vi "set_config_cluster.vi"(8 "error in (no error)":errorcluster, 10 "config cluster variant":variant, 11 "ClockDL090202FPGA in":refnum<class "ClockDL090202FPGA.lvclass">) -> (0 "error out":errorcluster, 3 "ClockDL090202FPGA out":refnum<class "ClockDL090202FPGA.lvclass">)   [LabVIEW 2010, in "ClockDL090202FPGA.lvclass"]
uses:
  ClockDL090202FPGA.lvclass
  ClockDL090202FPGA.lvclass/ClockDL090202FPGA.ctl
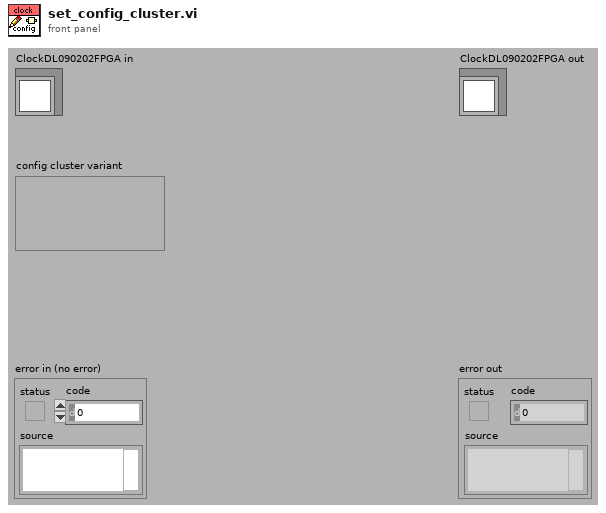
[diagram p1: front panel]
types:
  T1 = typedef "ClockDL090202FPGA.lvclass/config_data_cluster.ctl" = cluster{"FPGAWrapper":T2, "type":T3}
  T2 = typedef "plugin_specification.ctl" = cluster{"class path":string, "configuration":string, "label":string, "settings name":string}
  T3 = typedef "ClockDL090202FPGA.lvclass/type_enum.ctl" = enum16{"pixel clock", "gate 1", "gate 2", "gate 3"}
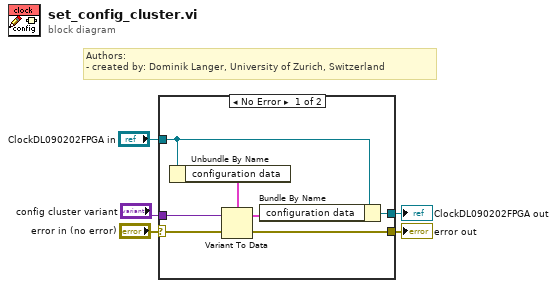
[diagram p0: block diagram]
diagram:
  # "Authors: \n- created by: Dominik Langer, University of Zurich, Switzerland"
  n1 = case shown="No Error" "error in (no error)" {
    selector: "error in (no error)" -> [w6 w14]
    tunnel: "config cluster variant" -> [w11 _]
    tunnel: "ClockDL090202FPGA in" -> [w10 w13]
    tunnel: [w8 w14] -> w3
    tunnel: [w7 w13] -> w2
    frame No Error {
      n2 = Unbundle By Name(w10) -> ("configuration data"=w12:T1)
      n3 = Variant To Data(error in=w6, Variant=w11, type=w12) -> (error out=w8:errorcluster, data=w9:T1)
      n4 = Bundle By Name(cluster=w10, "configuration data"=w9) -> (w7:refnum<class "ClockDL090202FPGA.lvclass">)
    }
    frame Error {
    }
  }
  "error out" <- w3
  "ClockDL090202FPGA out" <- w2
